vi "LVDimInterface.dis_add_command.vi"   [LabVIEW 2014, in "LVDimInterface.lvlib"]
doc: "Add a command to a DIM server. Whenever a new command is received by the server, the command data will be inserted into the LabVIEW event structure specified.\n\nImportant: One must call \"start serving\" to declare the new service to the dim name server.\n\nHistory: 16-DEC-2005, Dietrich Beck\n\nCopyright (C)\nGesellschaft für Schwerionenforschung, GSI\nPlanckstr. 1\n64291 Darmstadt\nGermany\n\nContact: D.Beck@gsi.de \n\nThis program is free software; you can redistribute it and/or modify it under the terms of the \nGNU General Public License as published by the Free Software Foundation; either version 2 of the license, or (at your option) any later version.\n\nThis program is distributed in the hope that it will be useful, but WITHOUT ANY WARRANTY; without even the implied warranty of MERCHANTABILITY or FITNESS FOR A PARTICULAR PURPOSE. See the GNU General License for more details (http://www.gnu.org).\n\nGesellschaft für Schwerionenforschung, GSI\nPlanckstr. 1, 64291 Darmstadt, Germany\nFor all questions and ideas contact D. Beck.\nLast update: 16-DEC-2005"
uses:
  LVDimInterface.lvlib
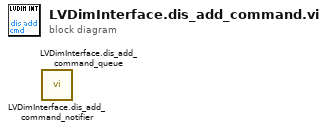
[diagram p0: block diagram]
diagram:
  n1 = call "LVDimInterface.dis_add_command_notifier.vi"() -> ()  [unwired: 18 in, 2 out]
  n2 = call "LVDimInterface.dis_add_command_queue.vi"() -> ()  [unwired: 18 in, 2 out]
